vi "Create_Unique_Array.vi"(11 "2D Array":dbl[][](array[numeric])) -> (1 "IJK indicies":i32[](array[numeric]), 3 "Unique Value Array":dbl[][](array[numeric]))   [LabVIEW 2011]
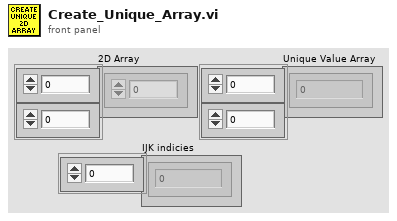
[diagram p1: front panel]
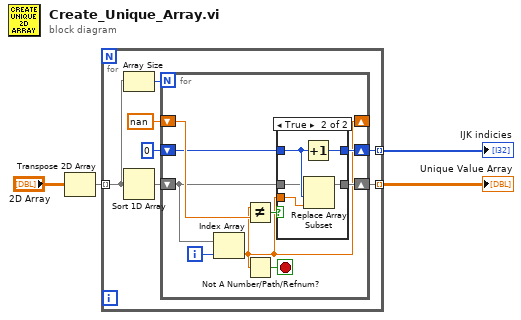
[diagram p0: block diagram]
diagram:
  n1 = Transpose 2D Array(2D array="2D Array") -> (transposed array=w4:dbl[][])
  n2 = for {
    tunnel: w4 -> [w7] mode=indexing
    tunnel: [w6] -> w3 mode=indexing
    tunnel: [w5] -> w1 mode=indexing
    n3 = Array Size(array=w7) -> (size(s)=w8:i32)
    n4 = Sort 1D Array(array=w7) -> (sorted array=w10:dbl[])
    n5 = for {
      N: w8 -> [_]
      shift-right: [w16] -> w5
      shift-left: w10 -> [w15]
      shift-right: [w12] -> _
      shift-left: nan ("Numeric 3") -> [w20]
      shift-right: [w17] -> w6
      shift-left: 0 -> [w18]
      i -> [w14]
      stop <- w13 stop-if-true
      n6 = Index Array(array=w15, index=w14) -> (element=w12:dbl)
      n7 = Not Equal?(x=w12, y=w20) -> (x != y?=w19:bool)
      n8 = Not A Number/Path/Refnum?(number/path/refnum=w12) -> (NaN/Path/Refnum?=w13:bool)
      n9 = case shown="True" w19 {
        tunnel: w18 -> [w22 w26]
        tunnel: [w22 w27] -> w17
        tunnel: w12 -> [_ w25]
        tunnel: w15 -> [w21 w24]
        tunnel: [w21 w23] -> w16
        frame False {
        }
        frame True {
          n10 = Increment(x=w26) -> (x+1=w27:i32)
          n11 = Replace Array Subset(array=w24, new element=w25, index=w26) -> (w23:dbl[])
        }
      }
    }
  }
  "IJK indicies" <- w3
  "Unique Value Array" <- w1
